vi "Auto1Bin.vi"(8 "error in":errorcluster) -> ()   [LabVIEW 2014]
uses:
  AutoLittleLessCheap.ctl
  <vilib>/Rock Robotics/WPI/DriverStation/WPI_DriverStationRobotMode2.ctl
  Robot Global Data.vi
  Gantry/GantryGlobals.vi
  AutomationGlobals.vi
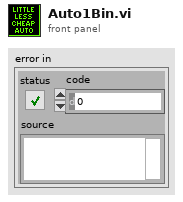
[diagram p1: front panel]
types:
  T1 = typedef "AutoLittleLessCheap.ctl" = enum16{"WaitingForInput", "FirstLift", "FirstOpenArms", "GantryOut", "Clamp", "Lift", "Strafe", "LowerLift", "OpenArms", "GantryIn"}
  T2 = typedef "WPI_DriverStationRobotMode2.ctl" = enum16{"Autonomous Disabled", "Autonomous Enabled", "Teleop Disabled", "Teleop Enabled", "Disconnected", "Finish", "Test Disabled", "Test Enabled", "Emergency Stopped"}
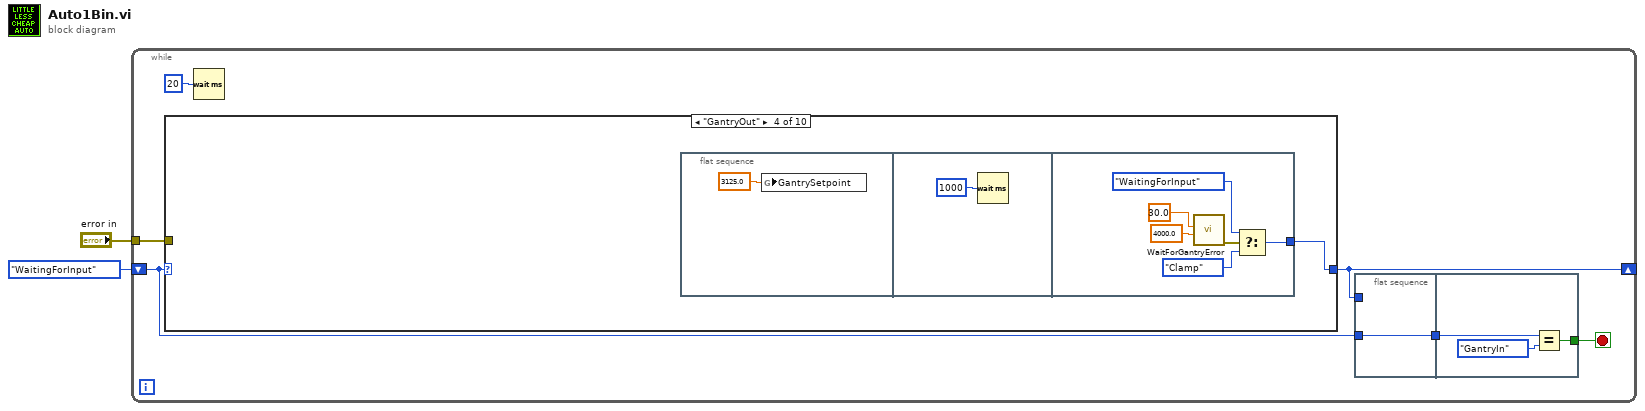
[diagram p0: block diagram]
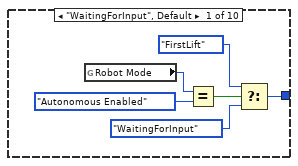
[diagram p2: hidden frame]
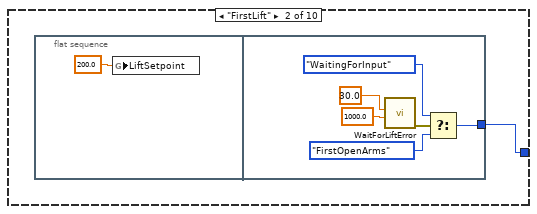
[diagram p3: hidden frame]
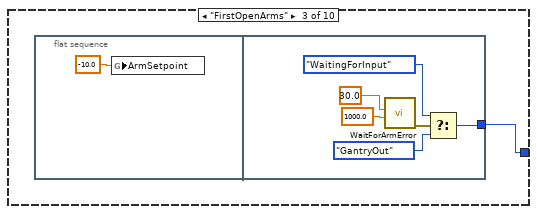
[diagram p4: hidden frame]
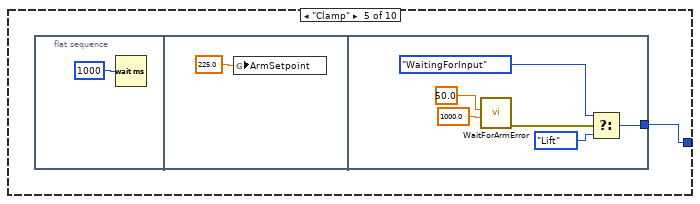
[diagram p5: hidden frame]
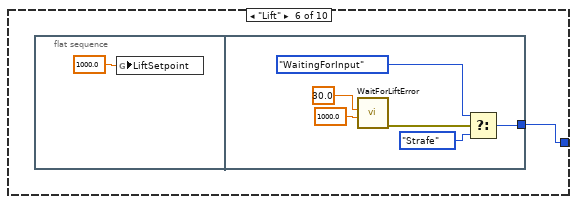
[diagram p6: hidden frame]
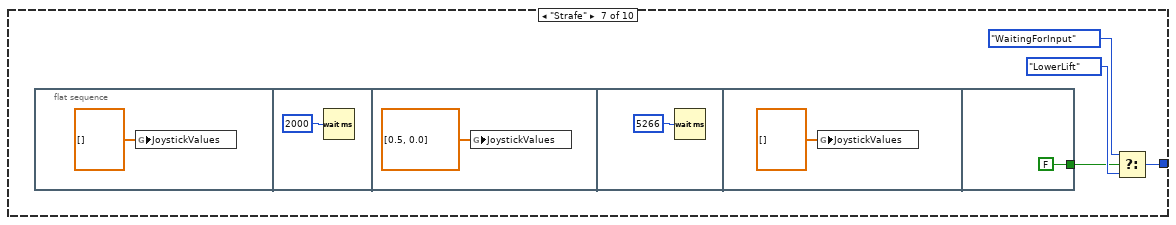
[diagram p7: hidden frame]
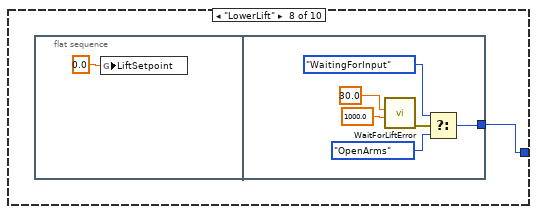
[diagram p8: hidden frame]
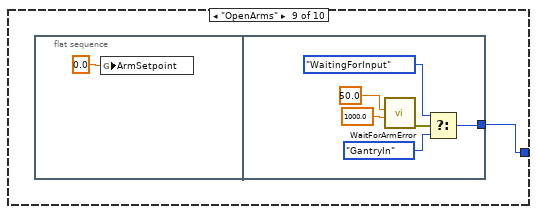
[diagram p9: hidden frame]
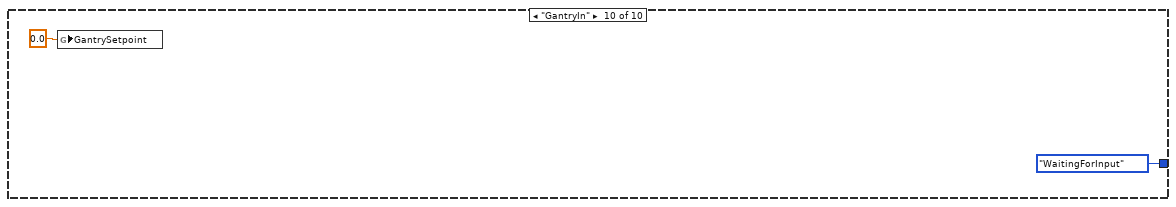
[diagram p10: hidden frame]
diagram:
  n1 = while {
    tunnel: "error in" -> [w8]
    shift-right: [w4] -> _
    shift-left: AutoLittleLessCheap."WaitingForInput" ("Auto") -> [w6]
    stop <- w7 stop-if-true
    n2 = case shown="\"GantryOut\"" w6 {
      tunnel: [w13 w19 w27 w35 w44 w53 w62 w71 w79 AutoLittleLessCheap."WaitingForInput" ("Auto")] -> w4
      tunnel: w8 -> [_ _ _ _ _ _ _ _ _ _]
      frame "WaitingForInput", Default {
        n3 = global read "Robot Global Data.vi" "Robot Mode"() -> (w18:T2)
        n4 = Equal?(x=w18, y=WPI_DriverStationRobotMode2."Autonomous Enabled") -> (x = y?=w16:bool)
        n5 = Select(t=AutoLittleLessCheap."FirstLift" ("Auto"), s=w16, f=AutoLittleLessCheap."WaitingForInput" ("Auto")) -> (s? t:f=w13:T1)
      }
      frame "FirstLift" {
        n6 = flat-sequence {
          tunnel: [w23] -> w19
          frame #0 {
            n7 = global write "GantryGlobals.vi" "LiftSetpoint"(200.0 ("LiftSetpoint")) -> ()
          }
          frame #1 {
            n8 = call "WaitForLiftError.vi"("Timeout (ms)"=1000.0, "AllowedError"=30.0) -> ("error out"=w26:errorcluster)  [unwired: 9 in]
            n9 = Select(t=AutoLittleLessCheap."WaitingForInput" ("Auto"), s=w26, f=AutoLittleLessCheap."FirstOpenArms" ("Auto")) -> (s? t:f=w23:T1)
          }
        }
      }
      frame "FirstOpenArms" {
        n10 = flat-sequence {
          tunnel: [w34] -> w27
          frame #0 {
            n11 = global write "GantryGlobals.vi" "ArmSetpoint"(-10.0 ("LiftSetpoint")) -> ()
          }
          frame #1 {
            n12 = call "WaitForArmError.vi"("Timeout (ms)"=1000.0, "AllowedError"=30.0) -> ("error out"=w33:errorcluster)  [unwired: 9 in]
            n13 = Select(t=AutoLittleLessCheap."WaitingForInput" ("Auto"), s=w33, f=AutoLittleLessCheap."GantryOut" ("Auto")) -> (s? t:f=w34:T1)
          }
        }
      }
      frame "GantryOut" {
        n14 = flat-sequence {
          tunnel: [w38] -> w35
          frame #0 {
            n15 = global write "GantryGlobals.vi" "GantrySetpoint"(3125.0 ("GantrySetpoint")) -> ()
          }
          frame #1 {
            n16 = Wait (ms)(milliseconds to wait=u32 1000) -> ()  [unwired: 1 out]
          }
          frame #2 {
            n17 = call "WaitForGantryError.vi"("Timeout (ms)"=4000.0, "AllowedError"=30.0) -> ("error out"=w41:errorcluster)  [unwired: 9 in]
            n18 = Select(t=AutoLittleLessCheap."WaitingForInput" ("Auto"), s=w41, f=AutoLittleLessCheap."Clamp" ("Auto")) -> (s? t:f=w38:T1)
          }
        }
      }
      frame "Clamp" {
        n19 = flat-sequence {
          tunnel: [w52] -> w44
          frame #0 {
            n20 = Wait (ms)(milliseconds to wait=u32 1000) -> ()  [unwired: 1 out]
          }
          frame #1 {
            n21 = global write "GantryGlobals.vi" "ArmSetpoint"(225.0 ("LiftSetpoint")) -> ()
          }
          frame #2 {
            n22 = call "WaitForArmError.vi"("Timeout (ms)"=1000.0, "AllowedError"=50.0) -> ("error out"=w51:errorcluster)  [unwired: 9 in]
            n23 = Select(t=AutoLittleLessCheap."WaitingForInput" ("Auto"), s=w51, f=AutoLittleLessCheap."Lift" ("Auto")) -> (s? t:f=w52:T1)
          }
        }
      }
      frame "Lift" {
        n24 = flat-sequence {
          tunnel: [w57] -> w53
          frame #0 {
            n25 = global write "GantryGlobals.vi" "LiftSetpoint"(1000.0 ("LiftSetpoint")) -> ()
          }
          frame #1 {
            n26 = call "WaitForLiftError.vi"("Timeout (ms)"=1000.0, "AllowedError"=30.0) -> ("error out"=w60:errorcluster)  [unwired: 9 in]
            n27 = Select(t=AutoLittleLessCheap."WaitingForInput" ("Auto"), s=w60, f=AutoLittleLessCheap."Strafe" ("Auto")) -> (s? t:f=w57:T1)
          }
        }
      }
      frame "Strafe" {
        n28 = flat-sequence {
          tunnel: [FALSE ("s")] -> w61
          frame #0 {
            n29 = global write "AutomationGlobals.vi" "JoystickValues"(dbl[] [] ("s? t:f")) -> ()
          }
          frame #1 {
            n30 = Wait (ms)(milliseconds to wait=u32 2000) -> ()  [unwired: 1 out]
          }
          frame #2 {
            n31 = global write "AutomationGlobals.vi" "JoystickValues"(dbl[] [0.5, 0.0] ("s? t:f")) -> ()
          }
          frame #3 {
            n32 = Wait (ms)(milliseconds to wait=u32 5266) -> ()  [unwired: 1 out]
          }
          frame #4 {
            n33 = global write "AutomationGlobals.vi" "JoystickValues"(dbl[] [] ("s? t:f")) -> ()
          }
          frame #5 {
          }
        }
        n34 = Select(t=AutoLittleLessCheap."WaitingForInput" ("Auto"), s=w61, f=AutoLittleLessCheap."LowerLift" ("Auto")) -> (s? t:f=w62:T1)
      }
      frame "LowerLift" {
        n35 = flat-sequence {
          tunnel: [w75] -> w71
          frame #0 {
            n36 = global write "GantryGlobals.vi" "LiftSetpoint"(0.0 ("LiftSetpoint")) -> ()
          }
          frame #1 {
            n37 = call "WaitForLiftError.vi"("Timeout (ms)"=1000.0, "AllowedError"=30.0) -> ("error out"=w78:errorcluster)  [unwired: 9 in]
            n38 = Select(t=AutoLittleLessCheap."WaitingForInput" ("Auto"), s=w78, f=AutoLittleLessCheap."OpenArms" ("Auto")) -> (s? t:f=w75:T1)
          }
        }
      }
      frame "OpenArms" {
        n39 = flat-sequence {
          tunnel: [w86] -> w79
          frame #0 {
            n40 = global write "GantryGlobals.vi" "ArmSetpoint"(0.0 ("LiftSetpoint")) -> ()
          }
          frame #1 {
            n41 = call "WaitForArmError.vi"("Timeout (ms)"=1000.0, "AllowedError"=50.0) -> ("error out"=w85:errorcluster)  [unwired: 9 in]
            n42 = Select(t=AutoLittleLessCheap."WaitingForInput" ("Auto"), s=w85, f=AutoLittleLessCheap."GantryIn" ("Auto")) -> (s? t:f=w86:T1)
          }
        }
      }
      frame "GantryIn" {
        n43 = global write "GantryGlobals.vi" "GantrySetpoint"(0.0 ("GantrySetpoint")) -> ()
      }
    }
    n44 = Wait (ms)(milliseconds to wait=u32 20) -> ()  [unwired: 1 out]
    n45 = flat-sequence {
      tunnel: w6 -> [w9]
      tunnel: [w9] -> w5
      tunnel: w4 -> [_]
      tunnel: [w11] -> w7
      tunnel: w5 -> [w10]
      frame #0 {
      }
      frame #1 {
        n46 = Equal?(x=w10, y=AutoLittleLessCheap."GantryIn" ("Auto")) -> (x = y?=w11:bool)
      }
    }
  }
